vi "Abort.vi"(8 "error in (no error)":errorcluster, 11 "VISA resource name":refnum<visa-resource-name>) -> (0 "error out":errorcluster, 3 "VISA resource name out":refnum<visa-resource-name>)   [LabVIEW 2017, in "Scope.lvlib" / "Tektronix DPO MSO 2000 4000 Series.lvlib"]
doc: "Aborts an acquisition and resets an oscilloscope to an idle state. \n<B>Note</B>: Only use this VI with other low-level VIs, such as the Initiate VI, the Fetch Waveform VI, and the Fetch Waveform Measurement VI. High-level VIs automatically incorporate the function of the Abort VI. This VI does not check the status of an instrument."
uses:
  Tektronix DPO MSO 2000 4000 Series.lvlib
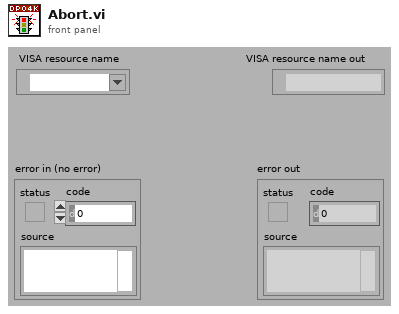
[diagram p1: front panel]
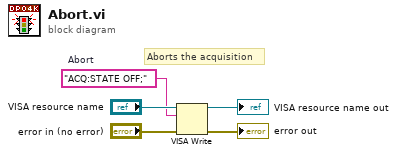
[diagram p0: block diagram]
diagram:
  w3 = "ACQ:STATE OFF;"  # Abort
  # "Aborts the acquisition"
  n1 = VISA Write(VISA resource name="VISA resource name", write buffer=w3, error in (no error)="error in (no error)") -> (VISA resource name out=→"VISA resource name out":refnum<visa-resource-name>, error out=→"error out":errorcluster)  [unwired: 1 out]
